vi "Set Shooter RPM.vi"(8 "Open Loop":bool, 9 "Increment":bool, 10 "Decrement":bool, 11 "Shooter Enabled":bool) -> ()   [LabVIEW 2011]
uses:
  System Set Points and States.vi
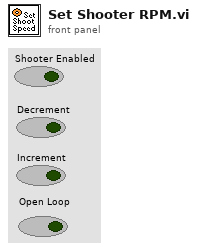
[diagram p1: front panel]
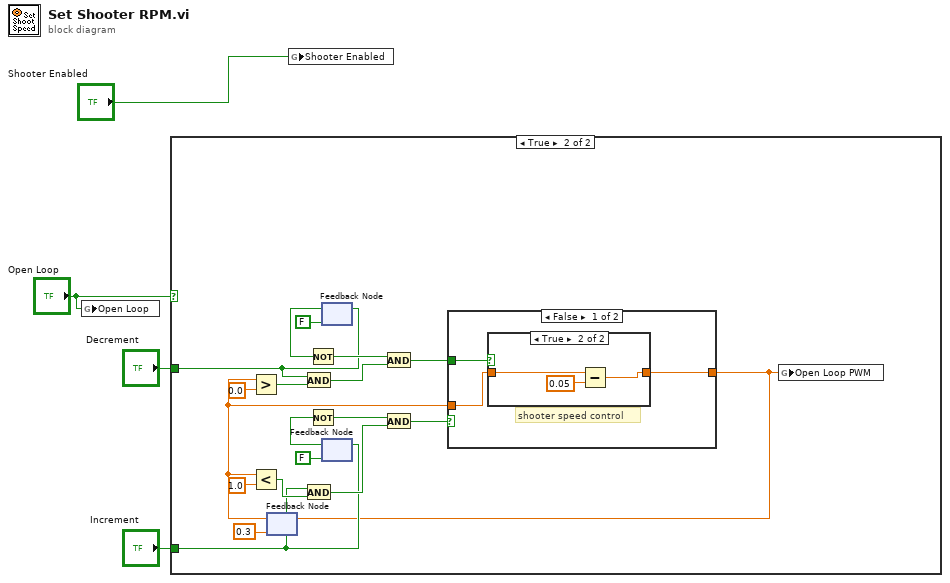
[diagram p0: block diagram]
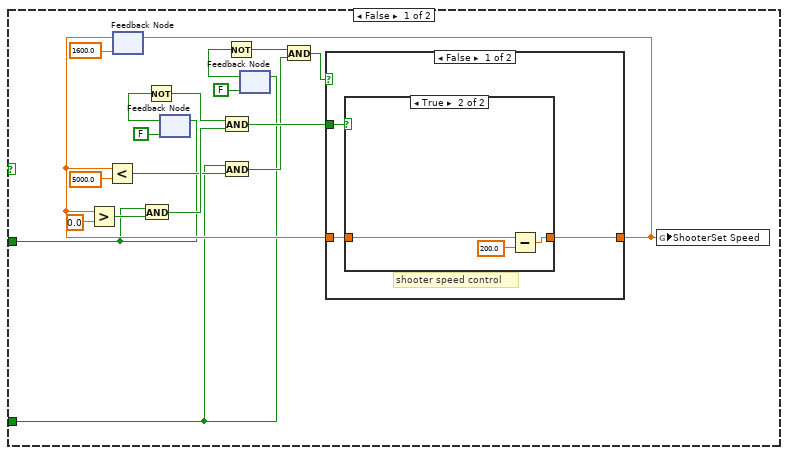
[diagram p2: hidden frame]
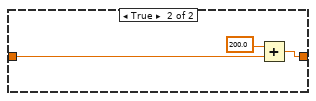
[diagram p4: hidden frame]
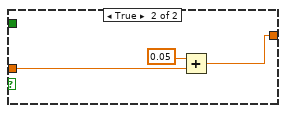
[diagram p6: hidden frame]
diagram:
  n1 = global write "System Set Points and States.vi" "Open Loop"("Open Loop") -> ()
  n2 = case shown="True" "Open Loop" {
    tunnel: "Decrement" -> [w6 w36]
    tunnel: "Increment" -> [w5 w35]
    frame False {
      n3 = feedback #1(1600.0) -> (w10:dbl)
      n4 = Greater?(x=w10, y=0.0) -> (0:w8:bool)
      n5 = Less?(x=w10, y=5000.0) -> (x < y?=w11:bool)
      n6 = And(x=w6, y=w8) -> (x .and. y?=w17:bool)
      n7 = feedback #2(FALSE) -> (w21:bool)
      n8 = Not(x=w21) -> (.not. x?=w22:bool)
      n9 = feedback-in #2(w6) -> ()
      n10 = And(x=w22, y=w17) -> (x .and. y?=w18:bool)
      n11 = And(x=w5, y=w11) -> (x .and. y?=w14:bool)
      n12 = feedback #3(FALSE) -> (w19:bool)
      n13 = Not(x=w19) -> (.not. x?=w20:bool)
      n14 = feedback-in #3(w5) -> ()
      n15 = And(x=w20, y=w14) -> (x .and. y?=w15:bool)
      n16 = case shown="False" w15 {
        tunnel: w18 -> [w26 _]
        tunnel: w10 -> [w25 w33]
        tunnel: [w24 w31] -> w7
        frame False {
          # "shooter speed control"
          n17 = case shown="True" w26 {
            tunnel: w25 -> [w27 w30]
            tunnel: [w27 w28] -> w24
            frame False {
            }
            frame True {
              n18 = Subtract(x=w30, y=200.0) -> (x-y=w28:dbl)
            }
          }
        }
        frame True {
          n19 = Add(x=200.0, y=w33) -> (x+y=w31:dbl)
        }
      }
      n20 = feedback-in #1(w7) -> ()
      n21 = global write "System Set Points and States.vi" "ShooterSet Speed"(w7) -> ()
    }
    frame True {
      n22 = feedback #4(0.3) -> (w39:dbl)
      n23 = Greater?(x=w39, y=0.0) -> (0:w52:bool)
      n24 = Less?(x=w39, y=1.0) -> (x < y?=w50:bool)
      n25 = And(x=w36, y=w52) -> (x .and. y?=w45:bool)
      n26 = And(x=w35, y=w50) -> (x .and. y?=w47:bool)
      n27 = feedback #5(FALSE) -> (w42:bool)
      n28 = Not(x=w42) -> (.not. x?=w41:bool)
      n29 = feedback-in #5(w36) -> ()
      n30 = feedback #6(FALSE) -> (w44:bool)
      n31 = Not(x=w44) -> (.not. x?=w43:bool)
      n32 = feedback-in #6(w35) -> ()
      n33 = And(x=w41, y=w45) -> (x .and. y?=w38:bool)
      n34 = And(x=w43, y=w47) -> (x .and. y?=w37:bool)
      n35 = case shown="False" w37 {
        tunnel: w38 -> [w55 _]
        tunnel: w39 -> [w54 w62]
        tunnel: [w53 w60] -> w34
        frame False {
          # "shooter speed control"
          n36 = case shown="True" w55 {
            tunnel: w54 -> [w56 w59]
            tunnel: [w56 w57] -> w53
            frame False {
            }
            frame True {
              n37 = Subtract(x=w59, y=0.05) -> (x-y=w57:dbl)
            }
          }
        }
        frame True {
          n38 = Add(x=0.05, y=w62) -> (x+y=w60:dbl)
        }
      }
      n39 = feedback-in #4(w34) -> ()
      n40 = global write "System Set Points and States.vi" "Open Loop PWM"(w34) -> ()
    }
  }
  n41 = global write "System Set Points and States.vi" "Shooter Enabled"("Shooter Enabled") -> ()
